vi "Open collector high-low control.vi"(8 "error in":errorcluster, 9 "TTL outputs":bool[](array[boolean]), 10 "Channels":string[](array[string]), 11 "Handle in":i32) -> (0 "error out":errorcluster, 3 "Handle out":i32)   [LabVIEW 2018]
panel:
  in  "Change?":bool
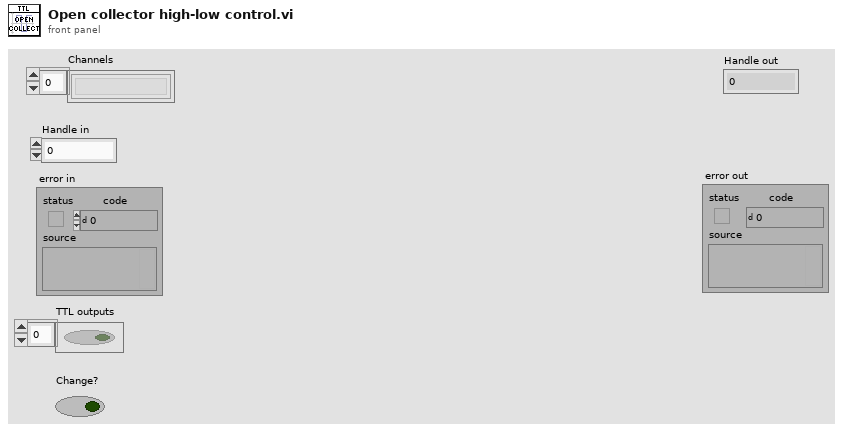
[diagram p1: front panel]
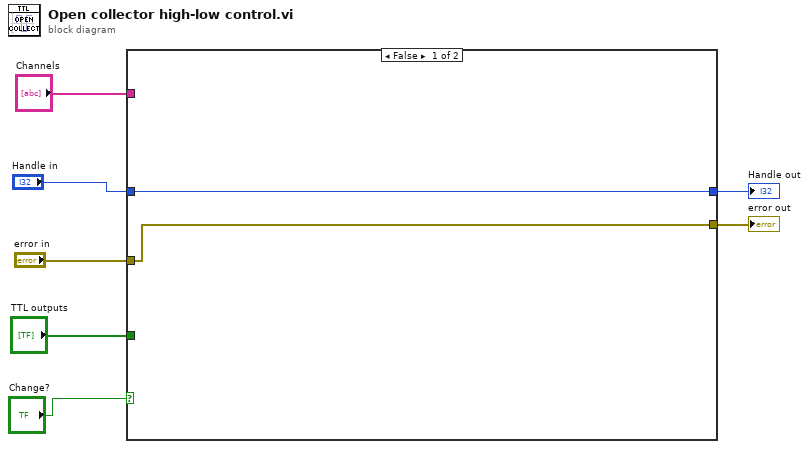
[diagram p0: block diagram]
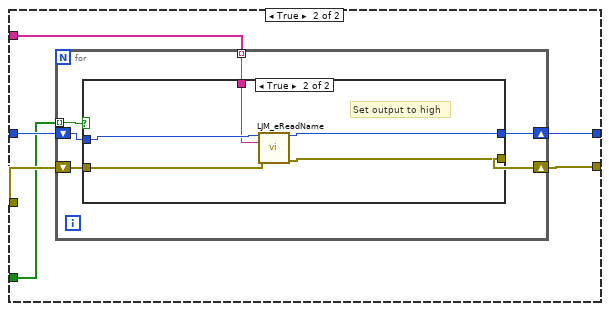
[diagram p2: hidden frame]
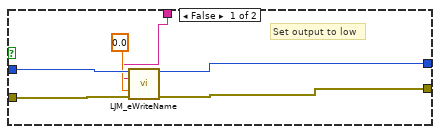
[diagram p3: hidden frame]
diagram:
  n1 = case shown="False" "Change?" {
    tunnel: "Channels" -> [_ w15]
    tunnel: "Handle in" -> [w8 w14]
    tunnel: "error in" -> [w9 w13]
    tunnel: [w8 w12] -> w4
    tunnel: [w9 w11] -> w3
    tunnel: "TTL outputs" -> [_ w10]
    frame False {
    }
    frame True {
      n2 = for {
        tunnel: w15 -> [w21] mode=indexing
        shift-right: [w18] -> w12
        shift-left: w14 -> [w20]
        shift-right: [w17] -> w11
        shift-left: w13 -> [w19]
        tunnel: w10 -> [w16] mode=indexing
        n3 = case shown="True" w16 {
          tunnel: w20 -> [w27 w32]
          tunnel: [w23 w29] -> w17
          tunnel: w19 -> [w26 w30]
          tunnel: [w24 w28] -> w18
          tunnel: w21 -> [w22 w31]
          frame False {
            # "Set output to low"
            n4 = call "LJM_eWriteName.vi"("Handle In"=w27, "Name"=w22, "Value"=0.0, "error in"=w26) -> ("Handle Out"=w24:i32, "error out"=w23:errorcluster)  [unwired: 10 in]
          }
          frame True {
            # "Set output to high"
            n5 = call "LJM_eReadName.vi"("Handle In"=w32, "Name"=w31, "error in"=w30) -> ("Handle Out"=w28:i32, "error out"=w29:errorcluster)  [unwired: 10 in, 1 out]
          }
        }
      }
    }
  }
  "Handle out" <- w4
  "error out" <- w3
